vi "(SubVI)Image_avging_FFT3_test.vi"(0 "buffer in":dbl[][](array[numeric]), 1 "index":dbl[](array[numeric]), 3 "Average":dbl min=0.0 max=1.0 step=0.01, 5 "data":dbl[][](array[numeric]), 7 "# of Cores":i32=3, 9 "input cluster":T1, 11 "error in (no error)":errorcluster, 12 "Soften Image":i32=1, 14 "power":dbl=0.01 min=0.01 max=1.0 step=0.01) -> (4 "buffer out":dbl[][](array[numeric]), 6 "Image":dbl[][](array[numeric]), 10 "complex_depth_profile":dbl[][](array[numeric]), 15 "error out":errorcluster)   [LabVIEW 2019]
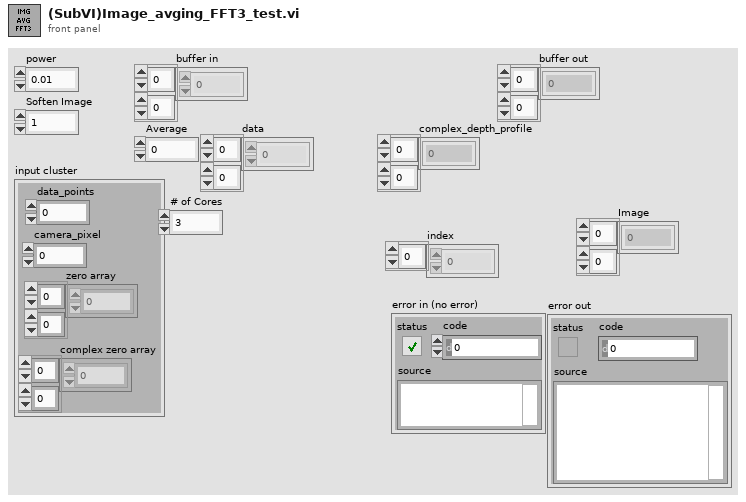
[diagram p1: front panel]
types:
  T1 = cluster{"data_points":i32, "camera_pixel":i32, "zero array":dbl[][], "complex zero array":dbl[][]}
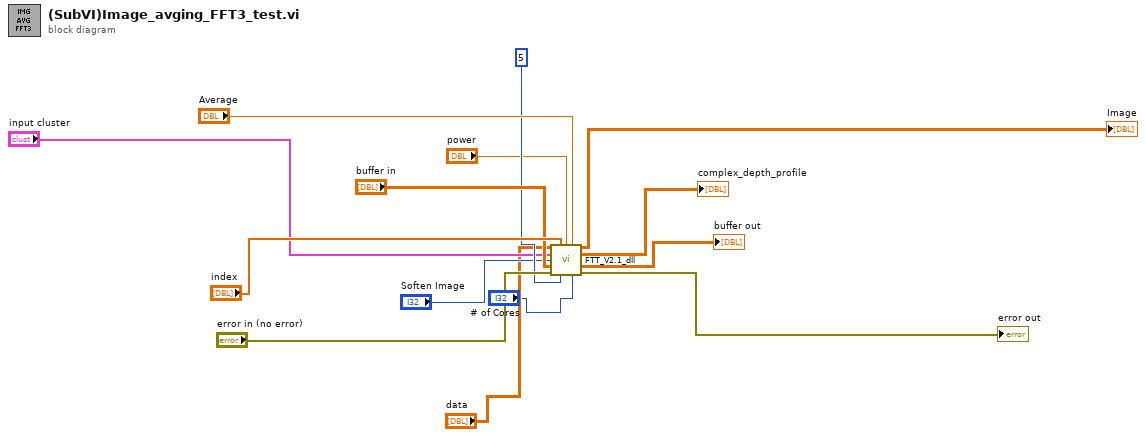
[diagram p0: block diagram]
diagram:
  n1 = call "FTT_V2.1_dll.vi"("data"="data", "index"="index", "power"="power", "alpha"="Average", "input cluster"="input cluster", "Blur_int"="Soften Image", "buffer in"="buffer in", "error in (no error)"="error in (no error)", "interp_value"=5, "# of Cores"="# of Cores") -> ("Depth_profile"=→"Image":dbl[][], "complex_depth_profile"=→"complex_depth_profile":dbl[][], "buffer out"=→"buffer out":dbl[][], "error out"=→"error out":errorcluster)  [unwired: 2 in]
